vi "Expansion_Permutation.vi"(1 "array":bool[](array[boolean])) -> (0 "Array":bool[](array[boolean]))   [LabVIEW 2013]
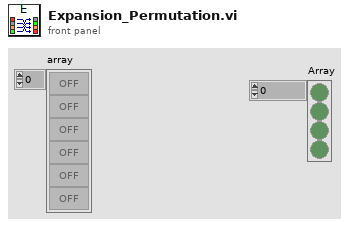
[diagram p1: front panel]
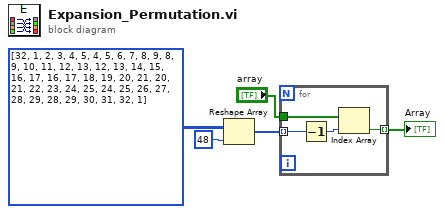
[diagram p0: block diagram]
diagram:
  n1 = Reshape Array(u8[][] [[32, 1, 2, 3, 4, 5], [4, 5, 6, 7, 8, 9], [8, 9, 10, 11, 12, 13], [12, 13, 14, 15, 16, 17], [16, 17, 18, 19, 20, 21], [20, 21, 22, 23, 24, 25], [24, 25, 26, 27, 28, 29], [28, 29, 30, 31, 32, 1]], 48 ("dimension size")) -> (w4:u8[])
  n2 = for {
    tunnel: "array" -> [w8]
    tunnel: w4 -> [w9] mode=indexing
    tunnel: [w6] -> w3 mode=indexing
    n3 = Decrement(x=w9) -> (x-1=w7:u8)
    n4 = Index Array(array=w8, index=w7) -> (element=w6:bool)
  }
  "Array" <- w3
